vi "Rotate.vi"(1 "Asynchronous":bool, 2 "Drive Speed":dbl, 3 "Drive Time":dbl) -> ()   [LabVIEW 2015]
doc: "This VI operates the robot's drive motors to rotate the robot for a specified time at a specified speed."
uses:
  <vilib>/Rock Robotics/WPI/Utilities/WPI_GetSetVariantRefNum.vi
  Robot Global Data.vi
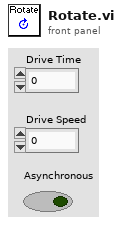
[diagram p1: front panel]
types:
  T1 = typedef "WPI_RobotDriveDevRef.ctl" = cluster{"DevStatus":errorcluster, "Motors[]":T2[], "Square Inputs":bool, "Max Output":dbl}
  T2 = typedef "WPI_MotorControlDeviceRef.ctl" = cluster{"DeviceStatus":errorcluster, "Type":T3, "PWM":cluster{"PWM Channel":T4, "DeadBand":T5}, "CAN":cluster{"Device Number":u8, "Control Mode":T6, "Semaphore":T7, "Max Vout":dbl, "TalonSRX Control Mode":T8}, "Invert":bool}
  T3 = typedef "WPI_MotorControlType.ctl" = enum16{"PWM", "CAN", "CANTalonSRX"}
  T4 = typedef "FPGA_DIOPWMChannel.ctl" = enum8{"PWM 0", "PWM 1", "PWM 2", "PWM 3", "PWM 4", "PWM 5", "PWM 6", "PWM 7", "PWM 8", "PWM 9", "PWM MXP 0", "PWM MXP 1", "PWM MXP 2", "PWM MXP 3", "PWM MXP 4", "PWM MXP 5", "PWM MXP 6", "PWM MXP 7", "PWM MXP 8", "PWM MXP 9", "Invalid"}
  T5 = typedef "WPI_PWMDeadband.ctl" = cluster{"Name":string, "maxPositivePwm":i32, "minPositivePwm":i32, "centerPwm":i32, "maxNegativePwm":i32, "minNegativePwm":i32, "angularRange":u16}
  T6 = typedef "WPI_CANJaguar_ControlMode.ctl" = enum8{"Percent VBus", "Current", "Speed", "Position", "Voltage"}
  T7 = typedef "Semaphore RefNum" = refnum<k1>
  T8 = typedef "WPI_CANTalonSRX_APIControlMode.ctl" = enum8{"Percent VBus", "Speed", "Position", "Slave", "Unchanged / Invalid", "Voltage Compensation", "Current", "Motion Profile"}
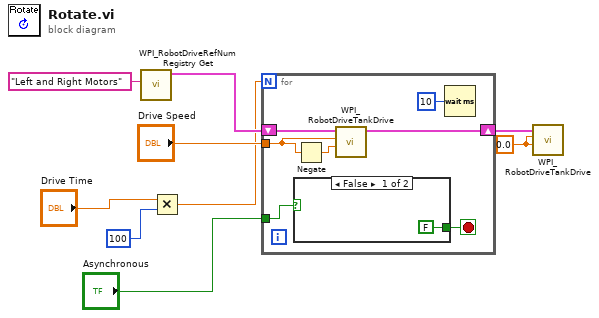
[diagram p0: block diagram]
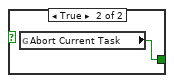
[diagram p2: hidden frame]
diagram:
  w2 = 0.0
  n1 = call <vilib>:"WPI_RobotDriveRefNum Registry Get.vi"("refnum name"="Left and Right Motors") -> ("RobotDriveDevRef"=w8:T1)  [unwired: 9 in, 1 out]
  n2 = Multiply(x="Drive Time", y=100) -> (x*y=w4:dbl)
  n3 = for {
    N: w4 -> [_]
    tunnel: "Drive Speed" -> [w13]
    shift-right: [w11] -> w3
    shift-left: w8 -> [w16]
    tunnel: "Asynchronous" -> [w10]
    stop <- w14 stop-if-true
    n4 = case shown="False" w10 {
      tunnel: [FALSE ("Abort Current Task") w18] -> w14
      frame False {
      }
      frame True {
        n5 = global read "Robot Global Data.vi" "Abort Current Task"() -> (w18:bool)
      }
    }
    n6 = Negate(x=w13) -> (-x=w12:dbl)
    n7 = call <vilib>:"WPI_RobotDriveTankDrive.vi"("Right axis value"=w12, "Left axis value"=w13, "RobotDriveDevRef"=w16) -> ("RobotDriveDevRef"=w11:T1)  [unwired: 6 in, 2 out]
    n8 = Wait (ms)(milliseconds to wait=u32 10) -> ()  [unwired: 1 out]
  }
  n9 = call <vilib>:"WPI_RobotDriveTankDrive.vi"("Right axis value"=w2, "Left axis value"=w2, "RobotDriveDevRef"=w3) -> ()  [unwired: 6 in, 3 out]
